vi "logic-train-sample-7-1-TEST-ALT.vi"() -> ()   [LabVIEW 2020]
uses:
  sample-7-1-state-enum.ctl
panel:
  in  "Request\nCapture":bool
  out "Hand_Close":bool
  out "Arm_Extend":bool
  out "State":T1
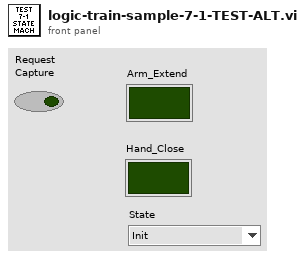
[diagram p1: front panel]
types:
  T1 = typedef "sample-7-1-state-enum.ctl" = enum16{"Init", "ExtendArm", "ExtendArmWait", "CloseHand", "CloseHandWait", "RetractArm", "RetractArmWait", "OpenHand", "OpenHandWait", "Ready"}
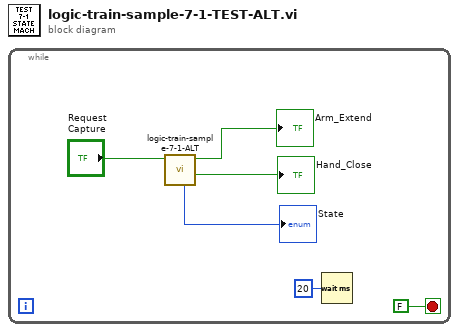
[diagram p0: block diagram]
diagram:
  n1 = while {
    stop <- FALSE stop-if-true
    n2 = call "logic-train-sample-7-1-ALT.vi"("Request\nCapture"="Request\nCapture") -> ("Hand_Close"=→"Hand_Close":bool, "Arm_Extend"=→"Arm_Extend":bool, "State"=→"State":T1)  [unwired: 8 in]
    n3 = Wait (ms)(milliseconds to wait=u32 20) -> ()  [unwired: 1 out]
  }
